vi "Read Parameters to process.vi"(8 "error in":errorcluster, 11 "Custom Controller Module runtime in":refnum<class "Custom Controller Module runtime.lvclass">) -> (0 "error out":errorcluster, 2 "Parameters to process":T1, 3 "Custom Controller Module runtime out":refnum<class "Custom Controller Module runtime.lvclass">)   [LabVIEW 2013, in "Custom Controller Module runtime.lvclass"]
uses:
  Custom Controller Module runtime.lvclass
  configuration/parameter data indices.ctl
  Custom Controller Module runtime.lvclass/Custom Controller Module runtime.ctl
  configuration/Custom Controller Module configuration.lvclass
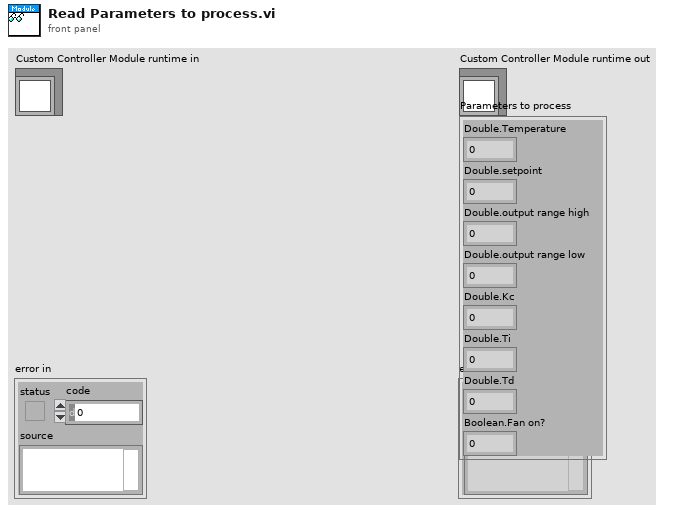
[diagram p1: front panel]
types:
  T1 = typedef "Custom Controller Module configuration.lvclass/parameter data indices.ctl" = cluster{"Double.Temperature":i32, "Double.setpoint":i32, "Double.output range high":i32, "Double.output range low":i32, "Double.Kc":i32, "Double.Ti":i32, "Double.Td":i32, "Boolean.Fan on?":i32}
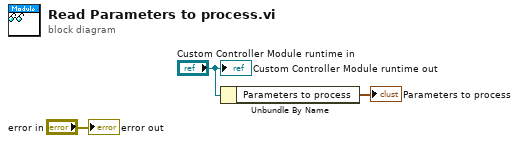
[diagram p0: block diagram]
diagram:
  n1 = Unbundle By Name("Custom Controller Module runtime in") -> ("Parameters to process"=→"Parameters to process":T1)
  "error out" <- "error in"
  "Custom Controller Module runtime out" <- "Custom Controller Module runtime in"
